vi "Write Experiment type.vi"(8 "error in (no error)":errorcluster, 10 "Experiment type":string, 11 "ActorMeter in":refnum<class "ActorMeter.lvclass">) -> (0 "error out":errorcluster, 3 "ActorMeter out":refnum<class "ActorMeter.lvclass">)   [LabVIEW 2014, in "ActorMeter.lvclass"]
uses:
  ActorMeter.lvclass
  ActorMeter.lvclass/ActorMeter.ctl
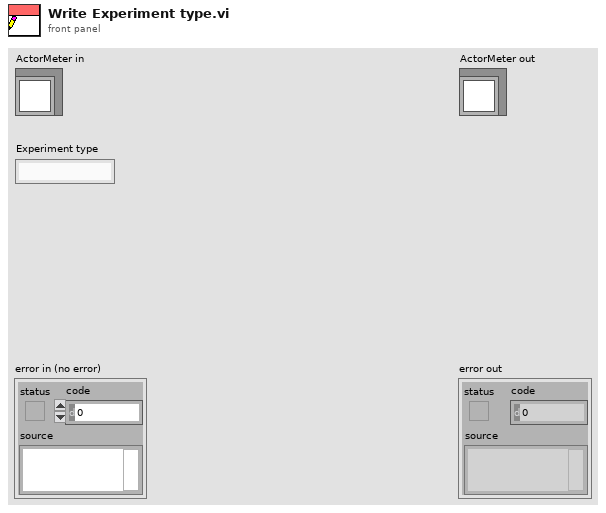
[diagram p1: front panel]
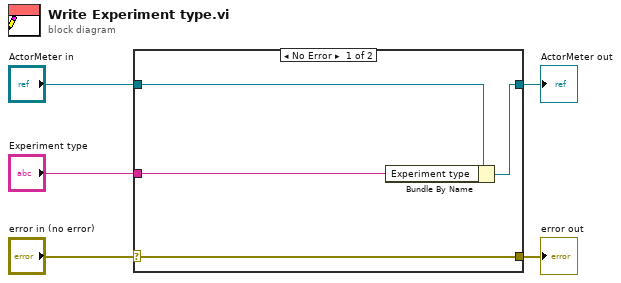
[diagram p0: block diagram]
diagram:
  n1 = case shown="No Error" "error in (no error)" {
    selector: "error in (no error)" -> [w9 w10]
    tunnel: [w9 w10] -> w4
    tunnel: [w7 w11] -> w2
    tunnel: "ActorMeter in" -> [w8 w11]
    tunnel: "Experiment type" -> [w6 _]
    frame No Error {
      n2 = Bundle By Name(cluster=w8, "Experiment type"=w6) -> (w7:refnum<class "ActorMeter.lvclass">)
    }
    frame Error {
    }
  }
  "error out" <- w4
  "ActorMeter out" <- w2
